vi "MainPannel.vi"() -> ()   [LabVIEW 2015]
uses:
  <vilib>/Utility/file.llb/Write Delimited Spreadsheet (I64).vi
  <vilib>/Utility/file.llb/Write Delimited Spreadsheet (DBL).vi
  <vilib>/express/express arith-compare/Formula/XNode/ExpressFormulaBlockNode.xnode
  <vilib>/LabVIEW Interface for Arduino/LabVIEW Interface for Arduino.lvlib
panel:
  out "Angle3":u8[](array[numeric])
  out "Angle2":i32[](array[numeric])
  out "Angle1":i32[](array[numeric])
  out "Angle 2 Microseconds Output":i32[](array[numeric])
  out "Angle1 Microseconds Output":i32[](array[numeric])
  out "Angle3 Output":u8[](array[numeric])
  out "State":bool
  out "Servo2 us":i32
  out "Servo1 us":i32
  out "X Check":dbl[](array[numeric])
  out "Y Check":dbl[](array[numeric])
  out "Angle3":u8=90
  out "Angle1":i32
  out "Angle 2":i32
  in  "Start Sketching":bool
  in  "Time Delay":dbl=1.0 caption="Delay Time (s)"
  out "Lift Array":bool[](array[boolean])
  out "Lift":bool
  out "Paint Image":picture
  out "# Points":i32
  out "Angle 1":dbl[](array[numeric])
  out "Angle 2":dbl[](array[numeric])
  out "Y Mapped":i32[](array[numeric])
  out "X Mapped":i32[](array[numeric])
  out "Index":i32[](array[numeric])
  out "Index":i32
  in  "Import a Picture":bool
  out "Array":bool[][](array[boolean])
  in  "path to JPEG file":path
  out "i":i32
  out "Replicate Y":i32[](array[numeric])
  out "Replicate X":i32[](array[numeric])
  out "Size(X)":i32
  out "Size (Y)":i32
  out "Y":i32[](array[numeric])
  out "X":i32[](array[numeric])
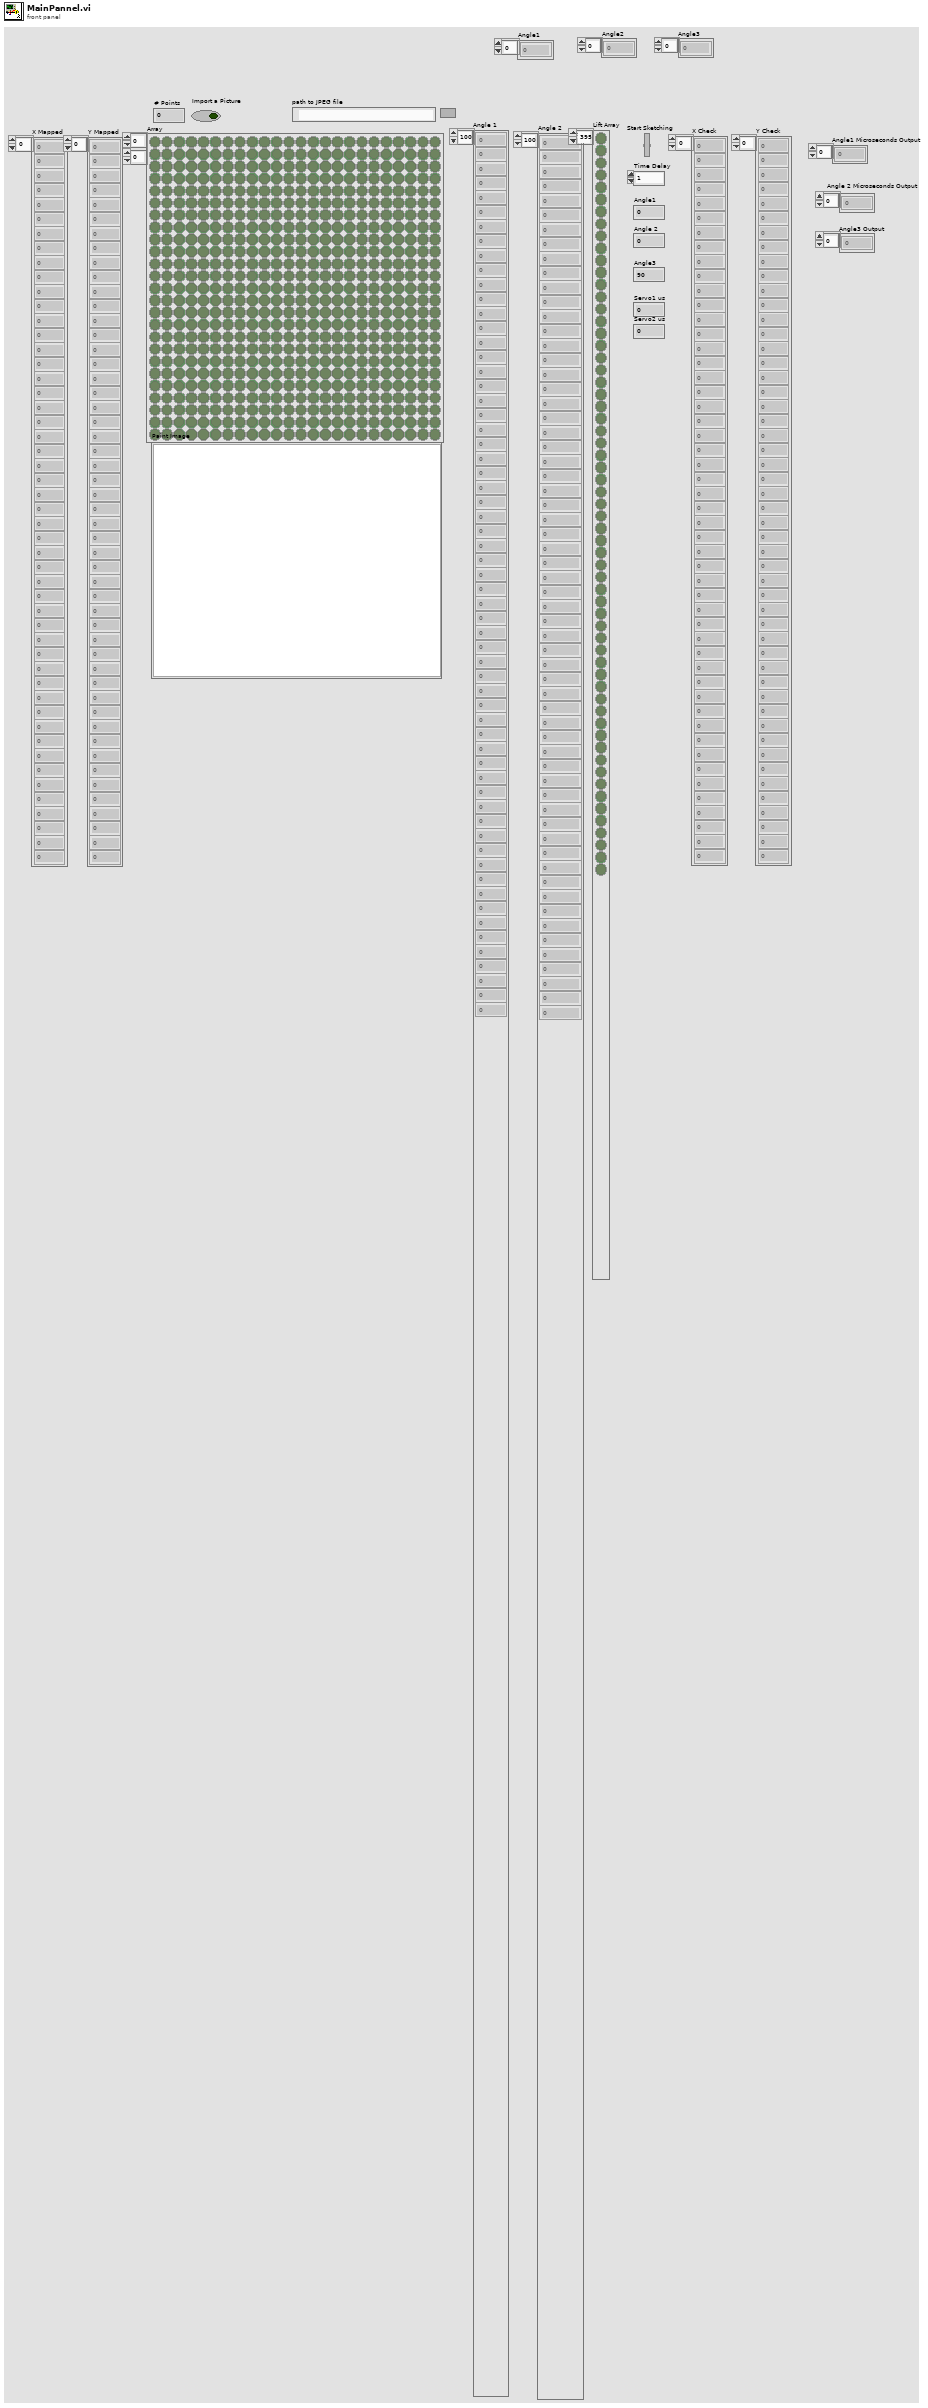
[diagram p1: front panel]
types:
  T1 = typedef "imagedata.ctl" = cluster{"image type":i32, "image depth":i32, "image":u8[], "mask":u8[], "colors":u32[], "Rectangle":cluster{"left":i16, "top":i16, "right":i16, "bottom":i16}}
  T2 = typedef "LabVIEW Interface for Arduino.lvlib/Arduino Resource.ctl" = cluster{"VISA resource":refnum<visa-resource-name>, "Board Type":T3, "Connection Type":enum8{"USB / Serial"}, "Bytes Per Packet (15)":u8}
  T3 = typedef "LabVIEW Interface for Arduino.lvlib/Board Type.ctl" = enum16{"Uno", "Dimuelanove w/Atmega 328", "Mega 2560"}
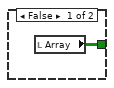
[diagram p2: hidden frame]
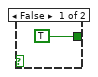
[diagram p3: hidden frame]
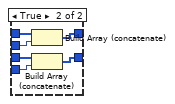
[diagram p4: hidden frame]
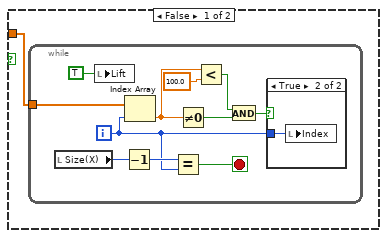
[diagram p5: hidden frame]
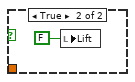
[diagram p7: hidden frame]
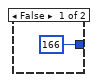
[diagram p8: hidden frame]
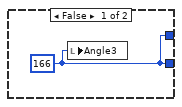
[diagram p10: hidden frame]
diagram:
  n1 = flat-sequence {
    tunnel: [w19] -> w14
    tunnel: [w52] -> w17
    tunnel: [w51] -> w16
    tunnel: [w50] -> w15
    tunnel: w14 -> [w49]
    tunnel: w17 -> [w62]
    tunnel: w16 -> [w60]
    tunnel: w15 -> [w58]
    tunnel: [w94] -> w13
    tunnel: w13 -> [w165]
    tunnel: [w163] -> w12
    tunnel: [w164] -> w11
    tunnel: [w163] -> w10
    tunnel: w12 -> [w200]
    tunnel: w11 -> [w199]
    tunnel: w10 -> [w198]
    tunnel: [w191] -> w9
    tunnel: [w191] -> w7
    tunnel: [w192] -> w5
    tunnel: [w191] -> w3
    tunnel: [w192] -> w2
    tunnel: [w191] -> w1
    tunnel: w9 -> [w286]
    tunnel: [w286] -> w8
    tunnel: w7 -> [w285]
    tunnel: [w285] -> w6
    tunnel: w5 -> [w284]
    tunnel: [w284] -> w4
    tunnel: w3 -> [w282]
    tunnel: w2 -> [w280]
    tunnel: w1 -> [w279]
    tunnel: w8 -> [w312]
    tunnel: w6 -> [w311]
    tunnel: w4 -> [w310]
    frame #0 {
      n2 = case shown="True" "Import a Picture" {
        tunnel: [w20 w23] -> w19
        frame False {
          n3 = local read "Array"() -> (w20:bool[][])
        }
        frame True {
          n4 = call <vilib>:"Read JPEG File.vi"("use 8 bit color table"=FALSE, "path to JPEG file"="path to JPEG file") -> ("image data"=w22:T1)  [unwired: 7 in, 2 out]
          n5 = call <vilib>:"Draw Flattened Pixmap.vi"("image data"=w22) -> ("new picture"=→"Paint Image":picture)  [unwired: 8 in]
          n6 = call <vilib>:"Unflatten Pixmap.vi"("image data"=w22) -> ("24-bit pixmap"=w30:u32[][])  [unwired: 4 in, 6 out]
          n7 = Matrix Size(0:w30) -> (1:w26:i32, 2:w27:i32)
          n8 = Decrement(x=w26) -> (x-1=w28:i32)
          n9 = Decrement(x=w27) -> (x-1=w29:i32)
          n10 = while {
            tunnel: w28 -> [w35]
            tunnel: w29 -> [w36]
            tunnel: w30 -> [w33]
            tunnel: [w31] -> w23 mode=indexing
            i -> [w32]
            stop <- w34 stop-if-true
            n11 = Equal?(x=w35, y=w32) -> (x = y?=w34:bool)
            n12 = while {
              tunnel: w36 -> [w46]
              tunnel: w33 -> [w44]
              tunnel: w32 -> [w43]
              tunnel: [w37] -> w31 mode=indexing
              i -> [w42]
              stop <- w45 stop-if-true
              n13 = Equal?(x=w46, y=w42) -> (x = y?=w45:bool)
              n14 = Index Array(array=w44, index (row)=w43, index (col)=w42) -> (element=w41:dbl)
              n15 = To Long Integer(number=w41) -> (32bit integer=w40:i32)
              n16 = Greater?(x=w40, y=10000000) -> (0:w38:bool)
              n17 = case shown="True" w38 {
                tunnel: [TRUE FALSE] -> w37
                frame False {
                }
                frame True {
                }
              }
            }
          }
        }
      }
    }
    frame #1 {
      n18 = Boolean To (0,1)(Boolean=w49) -> (0, 1=w50:i16[][])
      n19 = Matrix Size(0:w49) -> (1:w51:i32, 2:w52:i32)
      "Array" <- w49
    }
    frame #2 {
      n20 = Decrement(x=w60) -> (x-1=w59:i32)
      n21 = Decrement(x=w62) -> (x-1=w61:i32)
      n22 = while {
        tunnel: w61 -> [w70]
        tunnel: w59 -> [w69]
        tunnel: w58 -> [w68]
        tunnel: [w67] -> w55 mode=concatenating
        tunnel: [w64] -> w53 mode=concatenating
        i -> [w66]
        stop <- w71 stop-if-true
        n23 = Equal?(x=w69, y=w66) -> (x = y?=w71:bool)
        n24 = while {
          tunnel: w70 -> [w83]
          tunnel: w68 -> [w82]
          tunnel: w66 -> [w81]
          shift-right: [w77] -> w67
          shift-left: i32[] [] -> [w76]
          shift-right: [w73] -> w64
          shift-left: i32[] [] -> [w74]
          tunnel: w66 -> [w72]
          i -> [w75]
          stop <- w84 stop-if-true
          n25 = Equal?(x=w83, y=w75) -> (x = y?=w84:bool)
          n26 = Index Array(array=w82, index (row)=w81, index (col)=w75) -> (element=w80:dbl)
          n27 = Equal?(x=w80, y=1.0) -> (x = y?=w78:bool)
          n28 = case shown="False" w78 {
            tunnel: [w86 w92] -> w77
            tunnel: w76 -> [w86 w91]
            tunnel: w75 -> [_ w90]
            tunnel: w74 -> [w85 w89]
            tunnel: [w85 w88] -> w73
            tunnel: w72 -> [_ w87]
            frame False {
            }
            frame True {
              n29 = Build Array (concatenate)(w91, w90) -> (w92:i32[])
              n30 = Build Array (concatenate)(w89, w87) -> (w88:i32[])
            }
          }
        }
      }
      "X" <- w53
      "Y" <- w55
      "Replicate X" <- w53
      "Replicate Y" <- w55
      n31 = Array Size(array=w55) -> (size(s)=→"Size (Y)":i32)
      n32 = Array Size(array=w53) -> (size(s)=→"Size(X)":i32)
      "i" <- 0 ("i")
    }
    frame #3 {
      n33 = while {
        tunnel: [w97] -> w94 mode=indexing
        tunnel: [w95] -> w93 mode=indexing
        i -> [w100]
        stop <- w102 stop-if-true
        n34 = local read "Size(X)"() -> (w101:i32)
        n35 = flat-sequence {
          tunnel: [w103] -> w98
          tunnel: w98 -> [w126]
          tunnel: [w153] -> w96
          tunnel: [w162] -> w97
          tunnel: w96 -> [w162]
          tunnel: [w160] -> w95
          frame #0 {
            n36 = local read "Replicate X"() -> (w108:i32[])
            n37 = local read "Replicate Y"() -> (w107:i32[])
            n38 = local read "i"() -> (w104:i32)
            n39 = Index Array(array=w108, index=w104) -> (element=w106:i32)
            n40 = Index Array(array=w107, index=w104) -> (element=w105:i32)
            n41 = while {
              tunnel: w105 -> [w121]
              tunnel: w106 -> [w114]
              tunnel: w104 -> [_]
              tunnel: [w109] -> w103 mode=indexing
              i -> [w111]
              stop <- w110 stop-if-true
              n42 = local read "Size(X)"() -> (w113:i32)
              n43 = local read "Replicate X"() -> (w118:i32[])
              n44 = local read "Replicate Y"() -> (w116:i32[])
              n45 = Decrement(x=w113) -> (x-1=w112:i32)
              n46 = Equal?(x=w112, y=w111) -> (x = y?=w110:bool)
              n47 = Index Array(array=w118, index=w111) -> (element=w117:i32)
              n48 = Index Array(array=w116, index=w111) -> (element=w115:i32)
              n49 = Subtract(x=w117, y=w114) -> (x-y=w124:i32)
              n50 = Subtract(x=w115, y=w121) -> (x-y=w122:i32)
              n51 = Square(x=w124) -> (x^2=w123:i32)
              n52 = Square(x=w122) -> (x^2=w120:i32)
              n53 = Add(x=w123, y=w120) -> (x+y=w119:i32)
              n54 = Square Root(x=w119) -> (sqrt(x)=w109:dbl)
            }
          }
          frame #1 {
            n55 = Search 1D Array(1D array=w126, element=1.0, start index (0)=0) -> (index of element=w125:i32)
            "Index" <- w125
            n56 = Not Equal?(x=w125, y=-1) -> (x != y?=w127:bool)
            n57 = case shown="False" w127 {
              tunnel: w126 -> [w132 _]
              frame False {
                n58 = Square Root(x=2.0) -> (sqrt(x)=w135:dbl)
                n59 = Search 1D Array(1D array=w132, element=w135, start index (0)=0) -> (index of element=w131:i32)
                n60 = local write "Index"(w131) -> ()
                n61 = Not Equal?(x=w131, y=-1) -> (x != y?=w133:bool)
                n62 = case shown="True" w133 {
                  tunnel: w132 -> [w138 _]
                  frame False {
                    n63 = while {
                      tunnel: w138 -> [w146]
                      i -> [w145]
                      stop <- w147 stop-if-true
                      n64 = local read "Size(X)"() -> (w149:i32)
                      n65 = local write "Lift"(TRUE ("Lift")) -> ()
                      n66 = Decrement(x=w149) -> (x-1=w148:i32)
                      n67 = Index Array(array=w146, index=w145) -> (element=w141:dbl)
                      n68 = Equal?(x=w148, y=w145) -> (x = y?=w147:bool)
                      n69 = Not Equal To 0?(x=w141) -> (x != 0?=w142:bool)
                      n70 = Less?(x=w141, y=100.0) -> (x < y?=w143:bool)
                      n71 = And(x=w143, y=w142) -> (x .and. y?=w140:bool)
                      n72 = case shown="True" w140 {
                        tunnel: w145 -> [_ w150]
                        frame False {
                        }
                        frame True {
                          n73 = local write "Index"(w150) -> ()
                        }
                      }
                    }
                  }
                  frame True {
                    "Lift" <- FALSE ("Lift")
                  }
                }
              }
              frame True {
                n74 = local write "Lift"(FALSE ("Lift")) -> ()
              }
            }
          }
          frame #2 {
            n75 = local read "Replicate X"() -> (w154:i32[])
            n76 = local read "Replicate Y"() -> (w155:i32[])
            n77 = local read "i"() -> (w153:i32)
            n78 = Replace Array Subset(array=w154, new element=10000 ("new element/subarray"), index=w153) -> (w157:i32[])
            n79 = Replace Array Subset(array=w155, new element=10000 ("new element/subarray"), index=w153) -> (w156:i32[])
            n80 = local write "Replicate X"(w157) -> ()
            n81 = local write "Replicate Y"(w156) -> ()
          }
          frame #3 {
            n82 = local read "Index"() -> (w161:i32)
            n83 = local write "i"(w161) -> ()
            n84 = local read "Lift"() -> (w160:bool)
          }
        }
        n85 = Decrement(x=w101) -> (x-1=w99:i32)
        n86 = Equal?(x=w99, y=w100) -> (x = y?=w102:bool)
      }
      "Index" <- w94
      "Lift Array" <- w93
    }
    frame #4 {
      n87 = Array Size(array=w165) -> (size(s)=w169:i32)
      n88 = Decrement(x=w169) -> (x-1=w166:i32)
      n89 = while {
        tunnel: w166 -> [w183]
        shift-right: [w180] -> w164
        shift-left: i32[] [] -> [w181]
        tunnel: w165 -> [w171]
        shift-right: [w176] -> w163
        shift-left: i32[] [] -> [w175]
        i -> [w170]
        stop <- w182 stop-if-true
        n90 = Equal?(x=w170, y=w183) -> (x = y?=w182:bool)
        n91 = Index Array(array=w171, index=w170) -> (element=w172:i32)
        n92 = Index Array(array=w171, index=w170) -> (element=w177:i32)
        n93 = local read "X"() -> (w173:i32[])
        n94 = local read "Y"() -> (w178:i32[])
        n95 = Index Array(array=w173, index=w172) -> (element=w174:i32)
        n96 = Index Array(array=w178, index=w177) -> (element=w179:i32)
        n97 = Build Array (concatenate)(w175, w174) -> (w176:i32[])
        n98 = Build Array (concatenate)(w181, w179) -> (w180:i32[])
      }
      "Y Mapped" <- w164
      "X Mapped" <- w163
    }
    frame #5 {
      n99 = Array Size(array=w198) -> (size(s)=w202:i32)
      "# Points" <- w202
      n100 = Decrement(x=w202) -> (x-1=w201:i32)
      n101 = while {
        tunnel: w201 -> [w259]
        tunnel: w200 -> [w257]
        tunnel: w199 -> [w256]
        tunnel: [w214] -> w191 mode=indexing
        tunnel: [w213] -> w192 mode=indexing
        tunnel: [w224] -> w197 mode=indexing
        tunnel: [w219] -> w196 mode=indexing
        tunnel: [w203] -> w187 mode=indexing
        tunnel: [w204] -> w186 mode=indexing
        i -> [w255]
        stop <- w258 stop-if-true
        w239 = 100.0 ("x")
        n102 = Equal?(x=w259, y=w255) -> (x = y?=w258:bool)
        n103 = Index Array(array=w257, index=w255) -> (element=w251:i32)
        n104 = Index Array(array=w256, index=w255) -> (element=w252:i32)
        n105 = xnode "Formula"("X"=w251, "Y"=w252) -> ("Result"=w234:dbl)  [unwired: 1 in, 1 out]
        n106 = Divide(x=w252, y=w251) -> (x/y=w253:dbl)
        n107 = Square(x=w234) -> (x^2=w236:dbl)
        n108 = Inverse Tangent(1:w253) -> (0:w254:dbl)
        n109 = Subtract(x=1.0, y=w236) -> (x-y=w238:dbl)
        n110 = expression code="(x/pi)*180.0" "radians to degrees"(w254) -> (w250:dbl)
        n111 = Square Root(x=w238) -> (sqrt(x)=w235:dbl)
        n112 = Inverse Tangent (2 Input)(1:w234, 2:w235) -> (0:w233:dbl)
        n113 = expression code="(x/pi)*180.0" "radians to degrees"(w233) -> (w214:dbl)
        n114 = expression code="(x/180.0)*pi" "degrees to radians"(w214) -> (w247:dbl)
        n115 = expression code="(x/180.0)*pi" "degrees to radians"(w214) -> (w241:dbl)
        n116 = Sine(x=w247) -> (sin(x)=w246:dbl)
        n117 = Cosine(x=w241) -> (cos(x)=w231:dbl)
        n118 = Multiply(x=w239, y=w246) -> (x*y=w245:dbl)
        n119 = Multiply(x=w239, y=w231) -> (x*y=w242:dbl)
        n120 = Add(x=132.0, y=w242) -> (x+y=w244:dbl)
        n121 = Divide(x=w245, y=w244) -> (x/y=w240:dbl)
        n122 = Inverse Tangent(1:w240) -> (0:w248:dbl)
        n123 = expression code="(x/pi)*180.0" "radians to degrees"(w248) -> (w249:dbl)
        n124 = Subtract(x=w250, y=w249) -> (x-y=w213:dbl)
        n125 = Add(x=w213, y=w214) -> (x+y=w226:dbl)
        n126 = expression code="(x/180.0)*pi" "degrees to radians"(w213) -> (w217:dbl)
        n127 = expression code="(x/180.0)*pi" "degrees to radians"(w226) -> (w215:dbl)
        n128 = Multiply(x=w214, y=470.0) -> (x*y=w209:dbl)
        n129 = Multiply(x=w213, y=470.0) -> (x*y=w210:dbl)
        n130 = Divide(x=w209, y=9.0) -> (x/y=w206:dbl)
        n131 = Divide(x=w210, y=9.0) -> (x/y=w205:dbl)
        n132 = Sine(x=w217) -> (sin(x)=w218:dbl)
        n133 = Cosine(x=w217) -> (cos(x)=w227:dbl)
        n134 = Sine(x=w215) -> (sin(x)=w216:dbl)
        n135 = Cosine(x=w215) -> (cos(x)=w225:dbl)
        n136 = To Long Integer(number=w206) -> (32bit integer=w204:i32)
        n137 = To Long Integer(number=w205) -> (32bit integer=w203:i32)
        n138 = Multiply(x=132.0, y=w218) -> (x*y=w222:dbl)
        n139 = Multiply(x=132.0, y=w227) -> (x*y=w230:dbl)
        n140 = Multiply(x=100.0, y=w216) -> (x*y=w220:dbl)
        n141 = Multiply(x=100.0, y=w225) -> (x*y=w229:dbl)
        n142 = Add(x=w222, y=w220) -> (x+y=w219:dbl)
        n143 = Add(x=w230, y=w229) -> (x+y=w224:dbl)
      }
      "Angle 2" <- w191
      "Angle 1" <- w192
      "Y Check" <- w196
      "X Check" <- w197
      n144 = Build Array(w192, w191) -> (w190:dbl[][])
      n145 = Build Array(w187, w186) -> (w188:i32[][])
      n146 = call-poly <vilib>:"Write Delimited Spreadsheet.vi"("file path (dialog if empty)"=path "C:/Users/karim chamaa/Desktop/Steps", "2D data"=w188, "delimiter (\\t)"="," ("delimiter (\\t)")) -> ()  [unwired: 11 in, 2 out]
      n147 = call-poly <vilib>:"Write Delimited Spreadsheet.vi"("file path (dialog if empty)"=path "C:/Users/karim chamaa/Desktop/MatlabData", "format (%.3f)"="%.6f", "2D data"=w190, "delimiter (\\t)"="," ("delimiter (\\t)")) -> ()  [unwired: 10 in, 2 out]
      "State" <- TRUE ("State")
    }
    frame #6 {
      n148 = Array Size(array=w282) -> (size(s)=w283:i32)
      n149 = local read "Lift Array"() -> (w278:bool[])
      n150 = Decrement(x=w283) -> (x-1=w281:i32)
      n151 = while {
        tunnel: w281 -> [w306]
        tunnel: w280 -> [w303]
        tunnel: w279 -> [w302]
        tunnel: [w294] -> w275 mode=indexing
        tunnel: [w293] -> w274 mode=indexing
        tunnel: w278 -> [w292]
        tunnel: [w287] -> w270 mode=indexing
        i -> [w291]
        stop <- w305 stop-if-true
        n152 = Equal?(x=w306, y=w291) -> (x = y?=w305:bool)
        n153 = Index Array(array=w303, index=w291) -> (element=w301:dbl)
        n154 = Index Array(array=w302, index=w291) -> (element=w297:dbl)
        n155 = Index Array(array=w292, index=w291) -> (element=w289:bool)
        n156 = Equal?(x=TRUE, y=w289) -> (x = y?=w288:bool)
        n157 = Multiply(x=w297, y=10.0) -> (x*y=w296:dbl)
        n158 = Subtract(x=180.0, y=w301) -> (x-y=w300:dbl)
        n159 = case shown="True" w288 {
          tunnel: [u8 166 ("Servo Number") u8 180 ("Servo Number")] -> w287
          frame False {
          }
          frame True {
          }
        }
        n160 = Multiply(x=w300, y=10.0) -> (x*y=w295:dbl)
        n161 = To Long Integer(number=w295) -> (32bit integer=w294:i32)
        n162 = To Long Integer(number=w296) -> (32bit integer=w293:i32)
      }
      "Angle1" <- w275
      "Angle2" <- w274
      "Angle3" <- w270
      n163 = call-poly <vilib>:"Write Delimited Spreadsheet.vi"("file path (dialog if empty)"=path "C:/Users/karim chamaa/Desktop/Angle3", "1D data"=w270, "delimiter (\\t)"="," ("delimiter (\\t)")) -> ()  [unwired: 11 in, 2 out]
      n164 = Build Array(w275, w274) -> (w273:i32[][])
      n165 = call-poly <vilib>:"Write Delimited Spreadsheet.vi"("file path (dialog if empty)"=path "C:/Users/karim chamaa/Desktop/PropellerData", "2D data"=w273, "delimiter (\\t)"="," ("delimiter (\\t)")) -> ()  [unwired: 11 in, 2 out]
    }
    frame #7 {
      n166 = case shown="True" "Start Sketching" {
        tunnel: w312 -> [_ w330]
        tunnel: w311 -> [_ w329]
        tunnel: w310 -> [_ w328]
        frame False {
        }
        frame True {
          n167 = Array Size(array=w330) -> (size(s)=w331:i32)
          n168 = Decrement(x=w331) -> (x-1=w318:i32)
          n169 = call <vilib>:"Init.vi"("VISA resource"=refnum<visa-resource-name> "COM9") -> ("Arduino Resource"=w341:T2)  [unwired: 17 in, 1 out]
          n170 = call <vilib>:"Set Number of Servos.vi"("Arduino Resource"=w341, "Number Of Servos (1)"=u8 3) -> ("Arduino Resource"=w343:T2)  [unwired: 12 in, 1 out]
          n171 = call <vilib>:"Configure Servo.vi"("Arduino Resource"=w343, "Servo Number (0)"=u8 0, "DIO Pin (2)"=u8 3) -> ("Arduino Resource"=w335:T2)  [unwired: 11 in, 1 out]
          n172 = call <vilib>:"Configure Servo.vi"("Arduino Resource"=w335, "Servo Number (0)"=u8 1, "DIO Pin (2)"=u8 5) -> ("Arduino Resource"=w334:T2)  [unwired: 11 in, 1 out]
          n173 = call <vilib>:"Configure Servo.vi"("Arduino Resource"=w334, "Servo Number (0)"=u8 2, "DIO Pin (2)"=u8 6) -> ("Arduino Resource"=w323:T2)  [unwired: 11 in, 1 out]
          n174 = local read "Lift Array"() -> (w327:bool[])
          n175 = call <vilib>:"Servo Write Angle.vi"("Arduino Resource"=w323, "Servo Number"=u8 2, "Angle (Degrees)"=u8 0) -> ("Arduino Resource"=w322:T2)  [unwired: 11 in, 1 out]
          n176 = while {
            tunnel: w318 -> [w361]
            tunnel: w329 -> [w359]
            tunnel: w328 -> [w358]
            tunnel: w322 -> [w357]
            tunnel: w327 -> [w351]
            tunnel: [w354] -> w326
            tunnel: [w353] -> w325
            tunnel: [w352] -> w324
            tunnel: [w346] -> w319 mode=indexing
            tunnel: [w345] -> w315 mode=indexing
            tunnel: [w344] -> w314 mode=indexing
            i -> [w350]
            stop <- w360 stop-if-true
            n177 = Equal?(x=w350, y=w361) -> (x = y?=w360:bool)
            n178 = flat-sequence {
              tunnel: w350 -> [w377]
              tunnel: w359 -> [w376]
              tunnel: w358 -> [w375]
              tunnel: w357 -> [w368]
              tunnel: [w368] -> w355
              tunnel: [w367] -> w353
              tunnel: [w374] -> w352
              tunnel: [w363] -> w345
              tunnel: [w362] -> w344
              tunnel: [w394] -> w356
              tunnel: w355 -> [w394]
              tunnel: w356 -> [w403]
              tunnel: w349 -> [w397]
              tunnel: [w398] -> w348
              tunnel: [w396] -> w346
              tunnel: w348 -> [w408]
              tunnel: [w408] -> w347
              tunnel: [w410] -> w354
              tunnel: w347 -> [w410]
              frame #0 {
                n179 = Index Array(array=w376, index=w377) -> (element=w366:dbl)
                n180 = Index Array(array=w375, index=w377) -> (element=w365:dbl)
                n181 = xnode "Formula"("Angle"=w366) -> ("Result"=w370:dbl)  [unwired: 1 in, 1 out]
                n182 = xnode "Formula"("Angle"=w365) -> ("Result"=w372:dbl)  [unwired: 1 in, 1 out]
                n183 = To Long Integer(number=w366) -> (32bit integer=→"Angle 2":i32)
                n184 = To Long Integer(number=w365) -> (32bit integer=→"Angle1":i32)
                n185 = To Long Integer(number=w370) -> (32bit integer=w362:i32)
                "Servo2 us" <- w362
                n186 = To Long Integer(number=w372) -> (32bit integer=w363:i32)
                "Servo1 us" <- w363
                n187 = call <vilib>:"Servo Write Pulse Width.vi"("Arduino Resource"=w368, "Servo Number"=u8 1, "Pulse Width in uS"=w362) -> ("Arduino Resource"=w367:T2)  [unwired: 11 in, 1 out]
                n188 = call <vilib>:"Servo Write Pulse Width.vi"("Arduino Resource"=w368, "Servo Number"=u8 0, "Pulse Width in uS"=w363) -> ("Arduino Resource"=w374:T2)  [unwired: 11 in, 1 out]
              }
              frame #1 {
                n189 = call "Time Delay"("Delay Time (s)"="Time Delay") -> ()  [unwired: 10 in, 1 out]
              }
              frame #2 {
                n190 = Equal?(x=TRUE, y=w397) -> (x = y?=w400:bool)
                n191 = case shown="True" w400 {
                  tunnel: [w404 w405] -> w399
                  tunnel: [w404 w405] -> w396
                  frame False {
                    w404 = u8 166 ("Servo Number")
                    n192 = local write "Angle3"(w404) -> ()
                  }
                  frame True {
                    w405 = u8 180 ("Servo Number")
                    n193 = local write "State"(TRUE ("State")) -> ()
                    "Angle3" <- w405
                  }
                }
                n194 = call <vilib>:"Servo Write Angle.vi"("Arduino Resource"=w403, "Servo Number"=u8 2, "Angle (Degrees)"=w399) -> ("Arduino Resource"=w398:T2)  [unwired: 11 in, 1 out]
              }
              frame #3 {
                n195 = local read "State"() -> (w407:bool)
                n196 = case shown="True" w407 {
                  frame False {
                  }
                  frame True {
                    n197 = call "Time Delay2"() -> ()  [unwired: 11 in, 1 out]
                  }
                }
              }
              frame #4 {
                n198 = local write "State"(FALSE ("State")) -> ()
              }
            }
            n199 = Index Array(array=w351, index=w350) -> (element=w349:bool)
          }
          "Angle3 Output" <- w319
          "Angle1 Microseconds Output" <- w315
          "Angle 2 Microseconds Output" <- w314
          n200 = call <vilib>:"Close.vi"("Arduino Resource"=w326) -> ()  [unwired: 14 in, 1 out]
          n201 = call <vilib>:"Close.vi"("Arduino Resource"=w325) -> ()  [unwired: 14 in, 1 out]
          n202 = call <vilib>:"Close.vi"("Arduino Resource"=w324) -> ()  [unwired: 14 in, 1 out]
          n203 = Build Array(w315, w314) -> (w313:i32[][])
          n204 = call-poly <vilib>:"Write Delimited Spreadsheet.vi"("file path (dialog if empty)"=path "C:/Users/karim chamaa/Desktop/ArduinoData", "2D data"=w313, "delimiter (\\t)"="," ("delimiter (\\t)")) -> ()  [unwired: 11 in, 2 out]
        }
      }
    }
  }
